vi "UMLEditor ControlBusyDialog.vi"(1 "Title/StatusText":string, 2 "I-Value":i32, 5 "error in (no error)":errorcluster, 6 "Action(SendStatusMessage)":T1=enum."SendStatusMessage") -> (15 "Open":bool, 16 "AbortRequested":bool, 19 "error out":errorcluster)   [LabVIEW 2016]
uses:
  <resource>/Framework/Providers/Open_GDS/UML/UMLEditor/UMLEditor BusyDialogAction.ctl
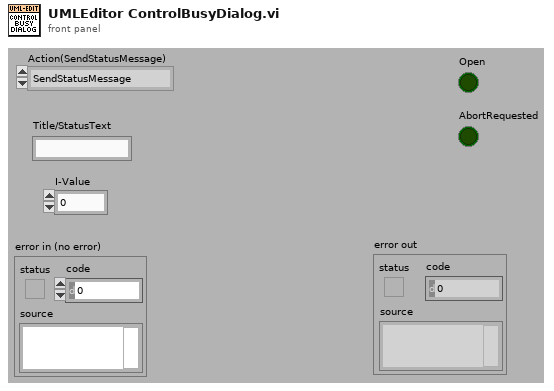
[diagram p1: front panel]
types:
  T1 = typedef "UMLEditor BusyDialogAction.ctl" = enum16{"Initialize", "Open(VIs)", "Open(i)", "Send_I-Value", "SendStatusMessage", "GetBusyDialogStatus", "Close", "Quit"}
  T2 = enum32{"Bad", "Idle", "Run top level", "Running"}
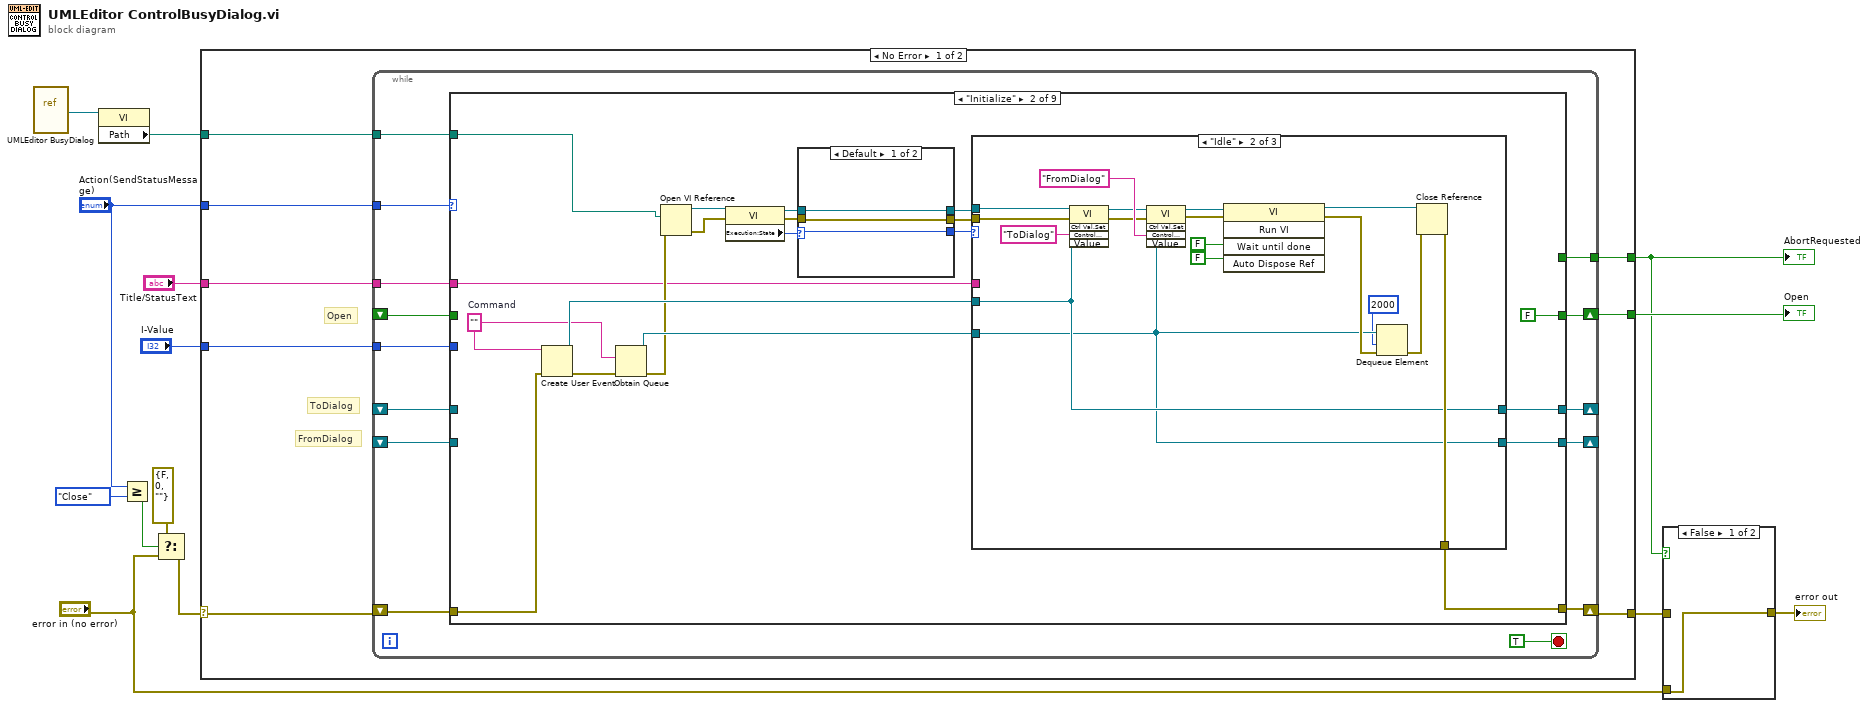
[diagram p0: block diagram]
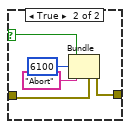
[diagram p2: hidden frame]
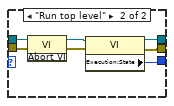
[diagram p4: hidden frame]
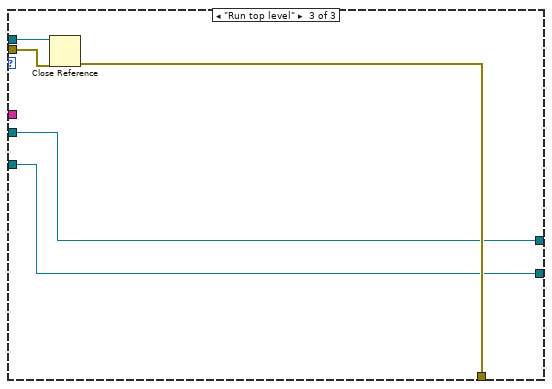
[diagram p6: hidden frame]
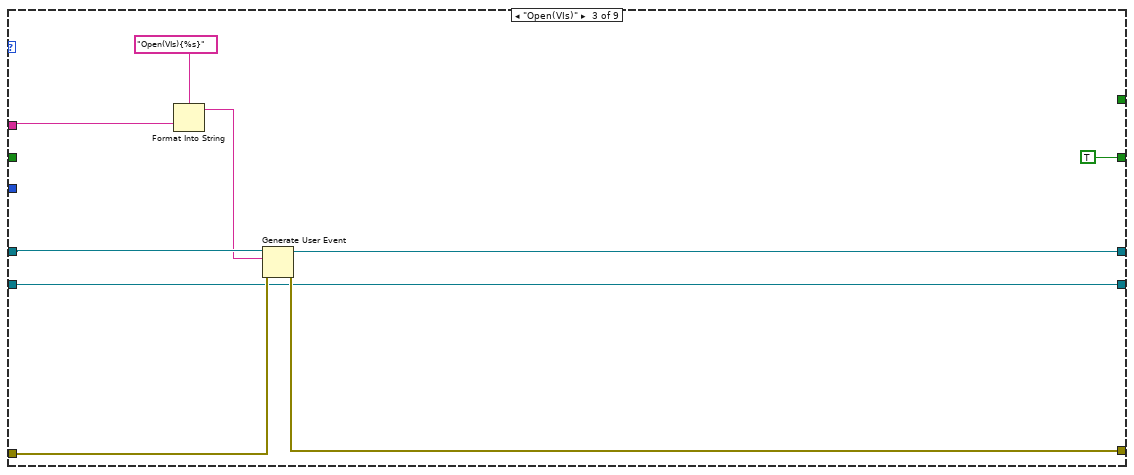
[diagram p7: hidden frame]
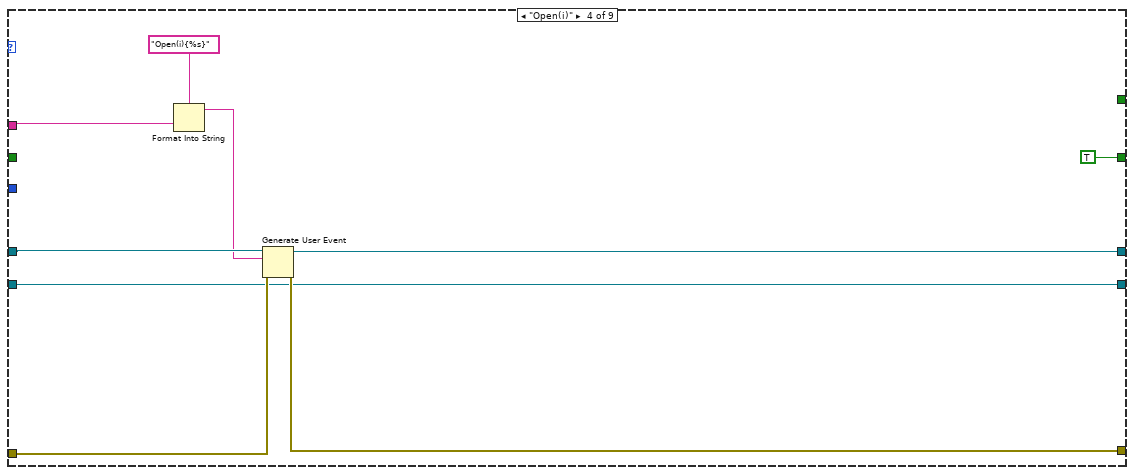
[diagram p8: hidden frame]
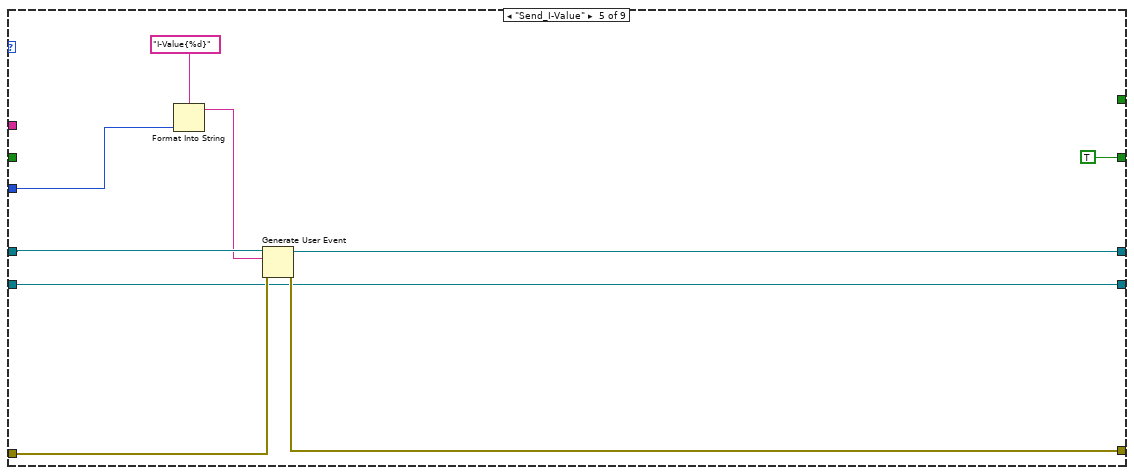
[diagram p9: hidden frame]
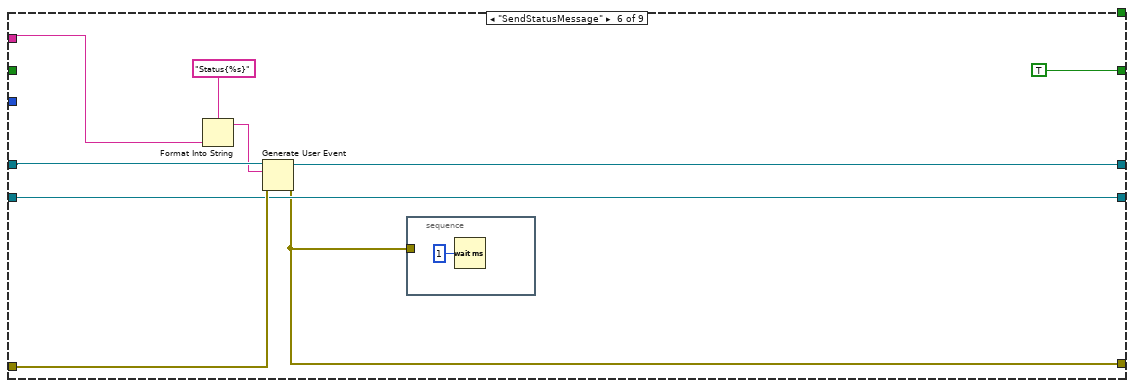
[diagram p10: hidden frame]
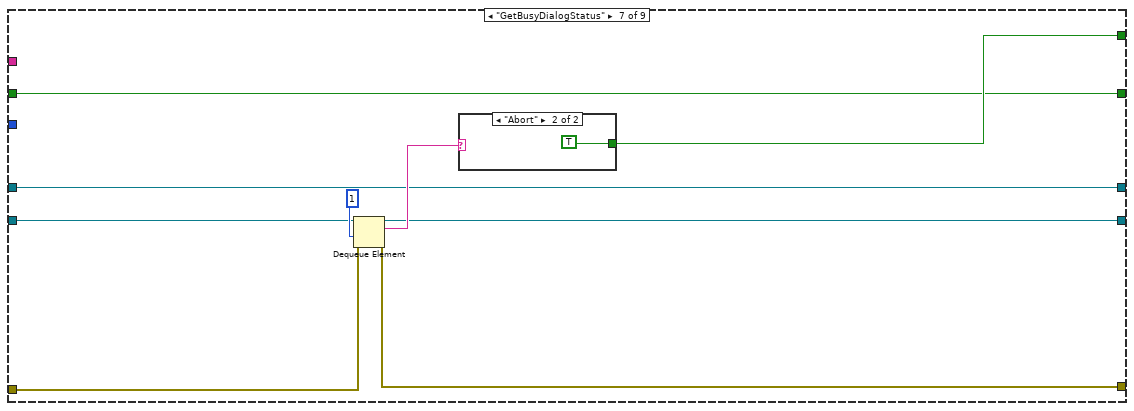
[diagram p11: hidden frame]
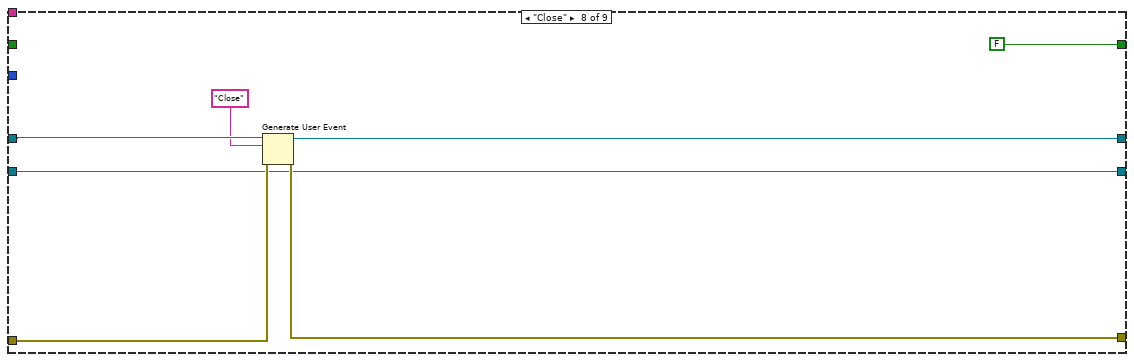
[diagram p13: hidden frame]
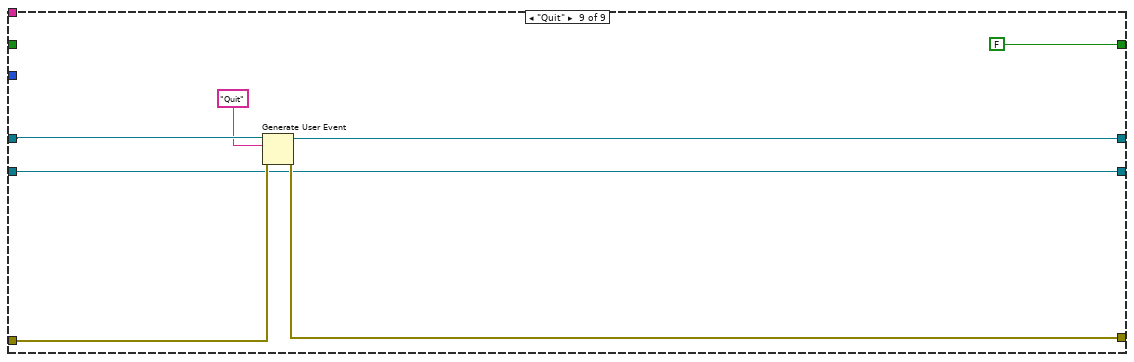
[diagram p14: hidden frame]
diagram:
  n1 = vi-ref <resource>:"UMLEditor BusyDialog.vi"() -> (w2:refnum<vi>)
  n2 = property class="VI"(reference=w2) -> ("Path"=w1:path)  [unwired: 1 in, 2 out]
  n3 = Greater Or Equal?(x="Action(SendStatusMessage)", y=UMLEditor_BusyDialogAction."Close") -> (x >= y?=w6:bool)
  n4 = Select(t=errorcluster {"status"=FALSE, "code"=0, "source"=""}, s=w6, f="error in (no error)") -> (s? t:f=w5:errorcluster)
  n5 = case shown="No Error" w5 {
    selector: w5 -> [w21 w157]
    tunnel: [w20 w157] -> w11
    tunnel: "Action(SendStatusMessage)" -> [w22 _]
    tunnel: "Title/StatusText" -> [w19 _]
    tunnel: [w18 _] -> w13
    tunnel: [w17 _] -> w12
    tunnel: "I-Value" -> [w16 _]
    tunnel: w1 -> [w15 _]
    frame No Error {
      # "Open"
      # "FromDialog"
      # "ToDialog"
      n6 = while {
        tunnel: w22 -> [w36]
        shift-right: [w34] -> w20
        shift-left: w21 -> [w35]
        shift-right: [w33] -> _
        shift-left: _ -> [w31]
        shift-right: [w32] -> _
        shift-left: _ -> [w30]
        tunnel: w19 -> [w28]
        shift-right: [w27] -> w18
        shift-left: _ -> [w26]
        tunnel: [w25] -> w17
        tunnel: w16 -> [w24]
        tunnel: w15 -> [w23]
        stop <- TRUE stop-if-true
        n7 = case shown="\"Initialize\"" w36 {
          tunnel: [w40 w60 w102 w111 w120 w123 w139 w147 w154] -> w34
          tunnel: w35 -> [w40 w59 w103 w112 w121 w130 w140 w148 w155]
          tunnel: [w39 w45 w101 w110 w119 w129 w133 w145 w152] -> w33
          tunnel: [w38 w44 w100 w109 w118 w128 w134 w144 w151] -> w32
          tunnel: w31 -> [w39 _ w104 w113 w122 w131 w133 w149 w156]
          tunnel: w30 -> [w38 _ w100 w109 w118 w128 w135 w144 w151]
          tunnel: w28 -> [_ w43 w97 w106 _ w126 _ _ _]
          tunnel: [w37 FALSE TRUE TRUE TRUE TRUE w136 FALSE FALSE] -> w27
          tunnel: w26 -> [w37 _ _ _ _ _ w136 _ _]
          tunnel: [_ _ _ _ _ _ w137 _ _] -> w25
          tunnel: w24 -> [_ _ _ _ w114 _ _ _ _]
          tunnel: w23 -> [_ w41 _ _ _ _ _ _ _]
          frame Default {
          }
          frame "Initialize" {
            w48 = ""  # Command
            n8 = Create User Event(user event datatype=w48, error in=w59) -> (user event=w50:refnum<user-event>, error out=w49:errorcluster)
            n9 = Obtain Queue(element data type=w48, error in (no error)=w49) -> (queue out=w47:refnum<queue>, error out=w46:errorcluster)  [unwired: 3 in, 1 out]
            n10 = Open VI Reference(vi path=w41, error in (no error)=w46) -> (vi reference=w58:refnum<vi>, error out=w57:errorcluster)  [unwired: 4 out]
            n11 = property class="VI"(reference=w58, error in=w57) -> (reference out=w56:refnum<vi>, error out=w55:errorcluster, "Execution:State"=w54:T2)
            n12 = case shown="Default" w54 {
              selector: w54 -> [w63 _]
              tunnel: w56 -> [w61 w70]
              tunnel: w55 -> [w62 w69]
              tunnel: [w63 w66] -> w53
              tunnel: [w62 w64] -> w52
              tunnel: [w61 w65] -> w51
              frame Default {
              }
              frame "Run top level" {
                n13 = invoke class="VI" method="Abort VI"(reference=w70, error in=w69) -> (reference out=w68:refnum<vi>, error out=w67:errorcluster)  [unwired: 1 in, 1 out]
                n14 = property class="VI"(reference=w68, error in=w67) -> (reference out=w65:refnum<vi>, error out=w64:errorcluster, "Execution:State"=w66:T2)
              }
            }
            n15 = case shown="\"Idle\"" w53 {
              tunnel: w51 -> [_ w89 w95]
              tunnel: w52 -> [w73 w88 w94]
              tunnel: w50 -> [w72 w80 w92]
              tunnel: [w73 w82 w93] -> w60
              tunnel: w47 -> [w71 w75 w91]
              tunnel: [w72 w80 w92] -> w45
              tunnel: [w71 w75 w91] -> w44
              tunnel: w43 -> [_ _ _]
              frame "Bad", Default {
              }
              frame "Idle" {
                n16 = invoke class="VI" method="Ctrl Val.Set"(reference=w89, error in=w88, "Control Name"="ToDialog", "Value"=w80) -> (reference out=w76:refnum<vi>, error out=w77:errorcluster)  [unwired: 1 in, 3 out]
                n17 = invoke class="VI" method="Ctrl Val.Set"(reference=w76, error in=w77, "Control Name"="FromDialog", "Value"=w75) -> (reference out=w79:refnum<vi>, error out=w78:errorcluster)  [unwired: 1 in, 3 out]
                n18 = invoke class="VI" method="Run VI"(reference=w79, error in=w78, "Wait until done"=FALSE, "Auto Dispose Ref"=FALSE) -> (reference out=w84:refnum<vi>, error out=w83:errorcluster)  [unwired: 1 in, 3 out]
                n19 = Dequeue Element(queue=w75, timeout in ms (-1)=2000, error in (no error)=w83) -> (error out=w90:errorcluster)  [unwired: 3 out]
                n20 = Close Reference(reference=w84, error in (no error)=w90) -> (error out=w82:errorcluster)
              }
              frame "Run top level" {
                n21 = Close Reference(reference=w95, error in (no error)=w94) -> (error out=w93:errorcluster)
              }
            }
          }
          frame "Open(VIs)" {
            n22 = Format Into String(format string="Open(VIs){%s}", w97) -> (resulting string=w96:string)  [unwired: 2 in, 1 out]
            n23 = Generate User Event(user event=w104, event data cluster=w96, error in=w103) -> (user event out=w101:refnum<user-event>, error out=w102:errorcluster)  [unwired: 1 in]
          }
          frame "Open(i)" {
            n24 = Format Into String(format string="Open(i){%s}", w106) -> (resulting string=w105:string)  [unwired: 2 in, 1 out]
            n25 = Generate User Event(user event=w113, event data cluster=w105, error in=w112) -> (user event out=w110:refnum<user-event>, error out=w111:errorcluster)  [unwired: 1 in]
          }
          frame "Send_I-Value" {
            n26 = Format Into String(format string="I-Value{%d}", w114) -> (resulting string=w115:string)  [unwired: 2 in, 1 out]
            n27 = Generate User Event(user event=w122, event data cluster=w115, error in=w121) -> (user event out=w119:refnum<user-event>, error out=w120:errorcluster)  [unwired: 1 in]
          }
          frame "SendStatusMessage" {
            n28 = Format Into String(format string="Status{%s}", w126) -> (resulting string=w124:string)  [unwired: 2 in, 1 out]
            n29 = Generate User Event(user event=w131, event data cluster=w124, error in=w130) -> (user event out=w129:refnum<user-event>, error out=w123:errorcluster)  [unwired: 1 in]
            n30 = stacked-sequence {
              tunnel: w123 -> [_]
              frame #0 {
                n31 = Wait (ms)(milliseconds to wait=u32 1) -> ()  [unwired: 1 out]
              }
            }
          }
          frame "GetBusyDialogStatus" {
            n32 = Dequeue Element(queue=w135, timeout in ms (-1)=1, error in (no error)=w140) -> (queue out=w134:refnum<queue>, element=w138:string, error out=w139:errorcluster)  [unwired: 1 out]
            n33 = case shown="\"Abort\"" w138 {
              tunnel: [_ TRUE] -> w137
              frame Default {
              }
              frame "Abort" {
              }
            }
          }
          frame "Close" {
            n34 = Generate User Event(user event=w149, event data cluster="Close" ("format string"), error in=w148) -> (user event out=w145:refnum<user-event>, error out=w147:errorcluster)  [unwired: 1 in]
          }
          frame "Quit" {
            n35 = Generate User Event(user event=w156, event data cluster="Quit" ("format string"), error in=w155) -> (user event out=w152:refnum<user-event>, error out=w154:errorcluster)  [unwired: 1 in]
          }
        }
      }
    }
    frame Error {
    }
  }
  "Open" <- w13
  "AbortRequested" <- w12
  n36 = case shown="False" w12 {
    selector: w12 -> [_ w161]
    tunnel: w11 -> [_ w163]
    tunnel: [w158 w162] -> w10
    tunnel: "error in (no error)" -> [w158 _]
    frame False {
    }
    frame True {
      n37 = Bundle(cluster=w163, "status"=w161, "code"=6100, "source"="Abort") -> (w162:errorcluster)
    }
  }
  "error out" <- w10
